vi "Main.vi"(11 "Module Admin":refnum<class "Delacor_lib_QMH_Module Admin.lvclass">) -> ()   [LabVIEW 2026, in "FT-818 CW Key Control.lvlib"]
doc: "This template is based off of the Queued Message Handler design pattern and the Queued Message Handler project template that ships with LabVIEW.\n\nThe main difference is that the queue is private to this module and communication between modules is performed via Broadcast and Request events.\n\nRequest events are wrapped in public API methods and are handled in the Event Handling Loop (EHL) of this VI. Any module can register for Broadcast events sent by this module. The EHL generates messages based on user interface actions.\n\nThe Message Handling Loop (MHL) processes messages generated by the EHL, or by other messages. The messages are string values, so new messages can be added easily to the Message Cases case structure in the MHL. Each message cluster can also provide an optional value for Message Data, which is a variant that can be converted to whatever message-specific data is required.\n_____\nBased on DQMH Dev Tools: Project Template 7.1.2.1547."
uses:
  FT-818 CW Key Control.lvlib
  <vilib>/Delacor/Delacor QMH/Libraries/Message Queue_class/Delacor_lib_QMH_Message Queue.lvclass/Delacor_lib_QMH_Message Queue.ctl
  <vilib>/Delacor/Delacor QMH/Libraries/Module Admin_class/Delacor_lib_QMH_Module Admin.lvclass/Delacor_lib_QMH_Module Admin.ctl
  <vilib>/Delacor/Delacor QMH/Libraries/Message Queue_class/Delacor_lib_QMH_Message Queue.lvclass
  Module Data--cluster.ctl
  <vilib>/Utility/miscctls.llb/LVPointTypeDef.ctl
  <vilib>/Delacor/Delacor QMH/Libraries/Message Queue_class/Delacor_lib_QMH_Enqueue Message (Single).vi
  Stop Argument--cluster.ctl
  <vilib>/Delacor/Delacor QMH/Libraries/Module Admin_class/Delacor_lib_QMH_Module Admin.lvclass
  Connect to radio (Reply Payload)--cluster.ctl
  Connect to radio Argument--cluster.ctl
  <vilib>/Instr/_visa.llb/VISA Configure Serial Port (Instr).vi
  Send CW Tone Argument--cluster.ctl
  Send CW Tone (Reply Payload)--cluster.ctl
  801ab31c-6d94-4327-a799-783b4abf15f8.vi
  0e38ebe7-76c1-4907-b289-0177e71b42e0.vi
panel:
  out "error out":errorcluster
  out "Status":string
  in  "Simulate MHL Error":bool
  in  "Simulate EHL Error":bool
  # "Other processes communicate with this Module via its Public API (wrappers for its Request Events).\n\nThis Module communicates with other processes via its Broadcast Events.\nAny process that wants to receive these messages can register for this module's Broadcast events."
  # "This template is for the DQMH framework. See the block diagram for more information on how to use this template."
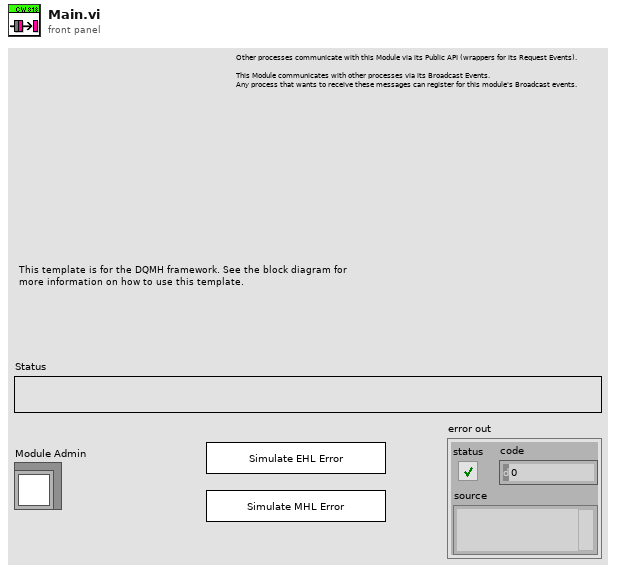
[diagram p1: front panel]
types:
  T1 = typedef "FT-818 CW Key Control.lvlib/Request Events--cluster.ctl" = cluster{"Stop Module":refnum<user-event>, "Show Panel":refnum<user-event>, "Hide Panel":refnum<user-event>, "Get Module Execution Status":refnum<user-event>, "Show Diagram":refnum<user-event>, "Connect to radio":refnum<user-event>, "Send CW Tone":refnum<user-event>}
  T2 = typedef "FT-818 CW Key Control.lvlib/Module Data--cluster.ctl" = cluster{"Status":string, "Radio Comm Port":refnum<visa-resource-name>}
  T3 = enum32{"invalid lock state", "Not Locked", "Locked (No Password)", "Password-protected"}
  T4 = typedef "FT-818 CW Key Control.lvlib/Stop Argument--cluster.ctl" = cluster{"Origin":string, "Exit via Stop Module Req?":bool, "Wait for Module to stop?":bool}
  T5 = typedef "FT-818 CW Key Control.lvlib/Connect to radio Argument--cluster.ctl" = cluster{"Radio Comm Port":refnum<visa-resource-name>, "CAT Rate":u32, "Wait Notifier":refnum<notifier>, "wait for reply":bool}
  T6 = typedef "FT-818 CW Key Control.lvlib/Send CW Tone Argument--cluster.ctl" = cluster{"CW Tone Time (ms)":u32, "Wait Notifier":refnum<notifier>, "wait for reply":bool}
  T7 = typedef "LVPointTypeDef.ctl" = cluster{"Horizontal":i16, "Vertical":i16}
  T8 = enum32{"Invalid", "Standard", "Closed", "Hidden", "Minimized", "Maximized"}
  T9 = typedef "FT-818 CW Key Control.lvlib/Connect to radio (Reply Payload)--cluster.ctl" = cluster{"Connected?":bool, "error":errorcluster}
  T10 = typedef "FT-818 CW Key Control.lvlib/Send CW Tone (Reply Payload)--cluster.ctl" = cluster{"error":errorcluster, "Done?":bool}
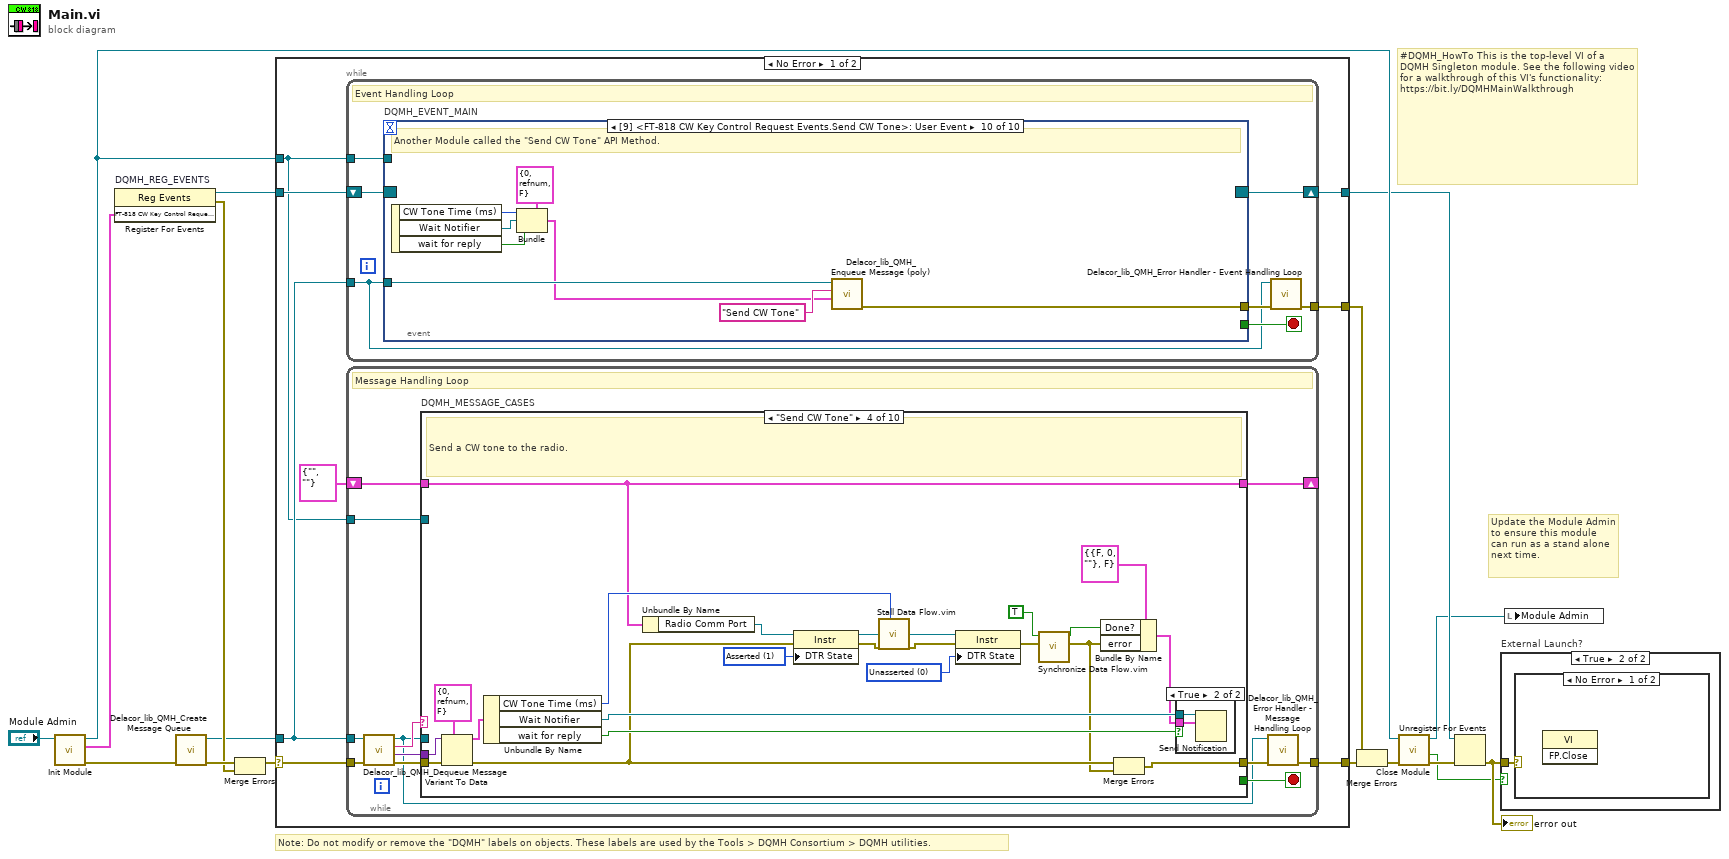
[diagram p0: block diagram]
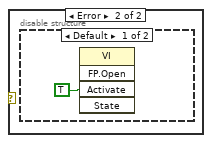
[diagram p3: hidden frame]
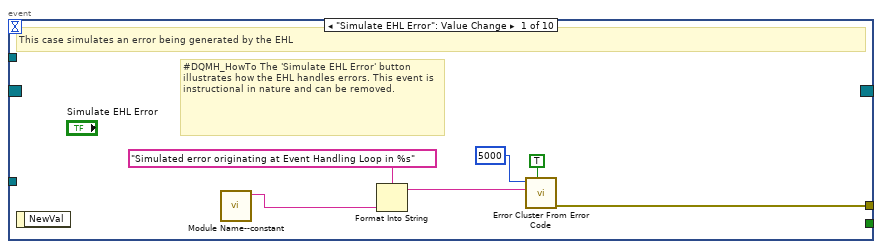
[diagram p5: hidden frame]
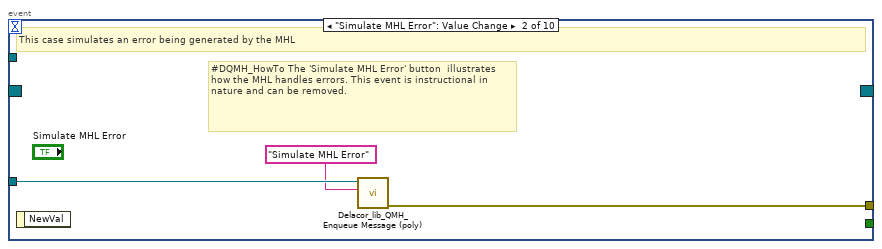
[diagram p6: hidden frame]
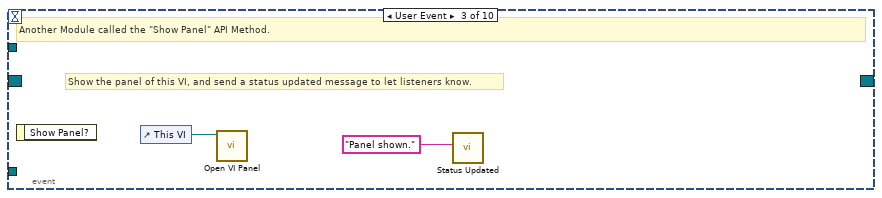
[diagram p7: hidden frame]
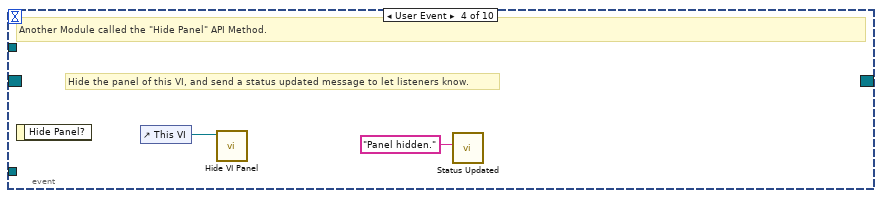
[diagram p8: hidden frame]
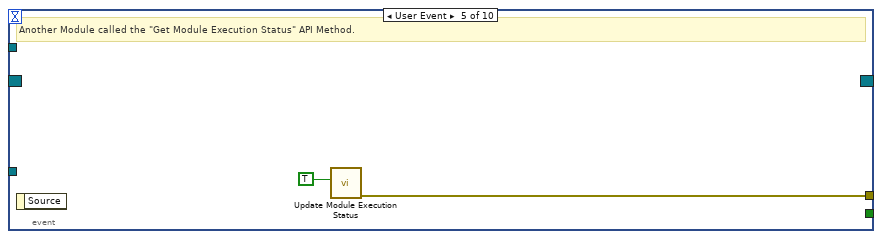
[diagram p9: hidden frame]
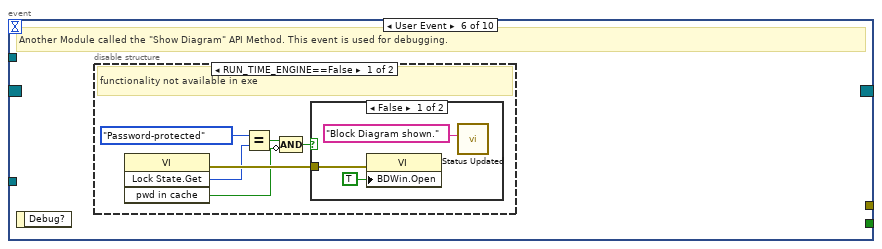
[diagram p10: hidden frame]
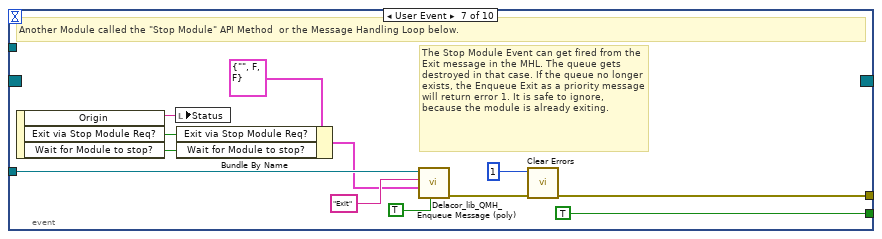
[diagram p13: hidden frame]
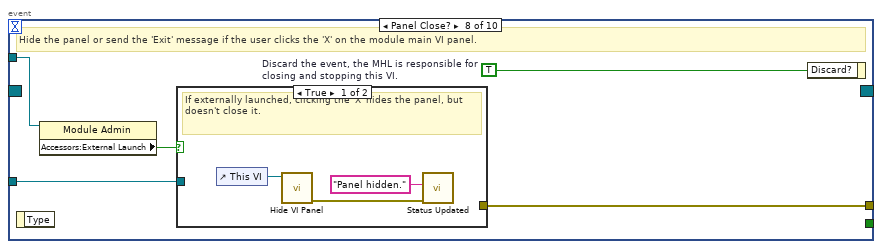
[diagram p14: hidden frame]
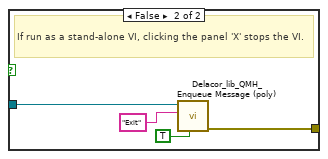
[diagram p15: hidden frame]
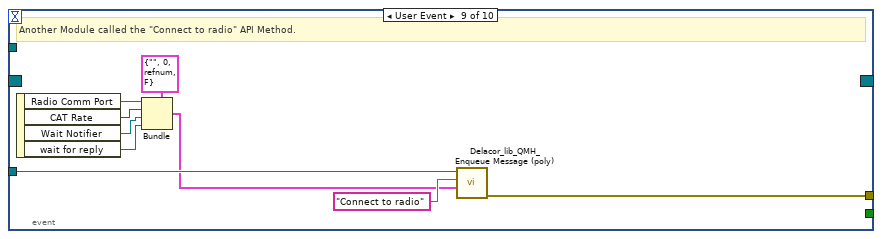
[diagram p16: hidden frame]
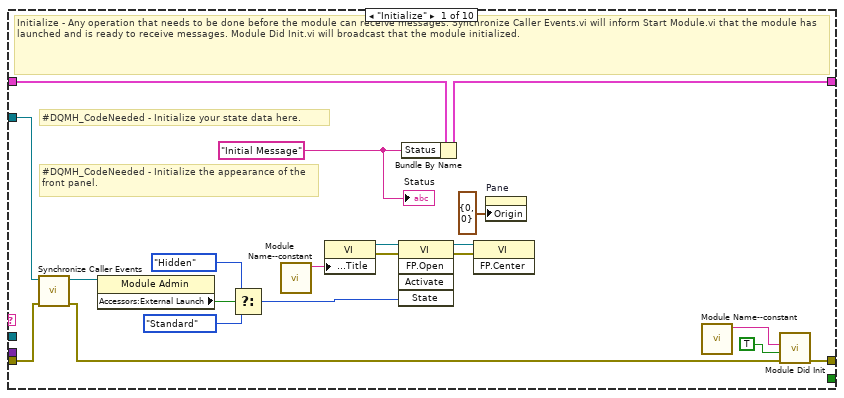
[diagram p17: hidden frame]
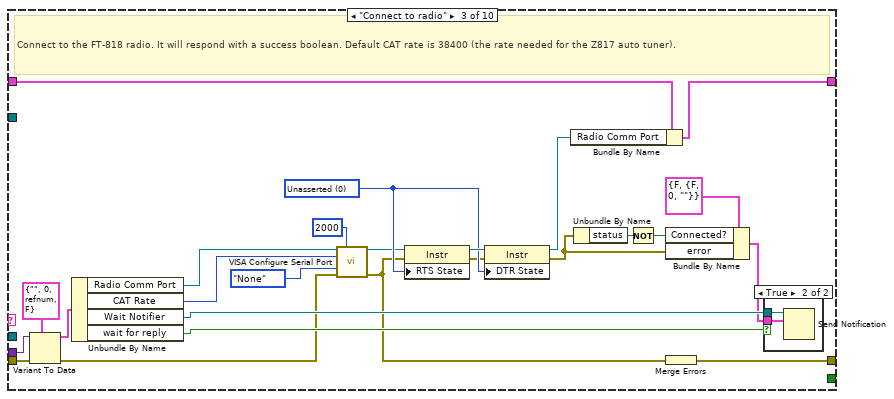
[diagram p19: hidden frame]
diagram:
  # "#DQMH_HowTo This is the top-level VI of a DQMH Singleton module. See the following video for a walkthrough of this VI's functionality: https://bit.ly/DQMHMainWalkthrough"
  # "Note: Do not modify or remove the \"DQMH\" labels on objects. These labels are used by the Tools > DQMH Consortium > DQMH utilities."
  # "Update the Module Admin to ensure this module can run as a stand alone next time."
  n1 = call "Init Module.vi"("Singleton Module Admin in"="Module Admin") -> ("error out"=w16:errorcluster, "FT-818 CW Key Control Request Events"=w5:T1, "Singleton Module Admin out"=w8:refnum<class "Delacor_lib_QMH_Module Admin.lvclass">)  [unwired: 8 in]
  n2 = register-events "DQMH_REG_EVENTS"(w5) -> (reference out=w6:refnum<event-registration>, error out=w9:errorcluster)  [unwired: 2 in]
  n3 = call <vilib>:"Delacor_lib_QMH_Create Message Queue.vi"("error in"=w16) -> ("error out"=w11:errorcluster, "Message Queue"=w4:refnum<class "Delacor_lib_QMH_Message Queue.lvclass">)  [unwired: 9 in]
  n4 = Merge Errors(w11, w9) -> (w10:errorcluster)
  n5 = case shown="No Error" w10 {
    selector: w10 -> [w23 w248]
    tunnel: [w25 w247] -> w17
    tunnel: [w22 w246] -> w7
    tunnel: w6 -> [w20 w246]
    tunnel: w4 -> [w19 w241]
    tunnel: [w24 _] -> w14
    tunnel: w8 -> [w18 w242]
    frame No Error {
      n6 = while {
        tunnel: w19 -> [w26]
        shift-right: [w29] -> w22
        shift-left: w20 -> [w30]
        tunnel: [w31] -> w24
        tunnel: w18 -> [w27]
        stop <- w28 stop-if-true
        # "Event Handling Loop"
        n7 = event "DQMH_EVENT_MAIN" shown="[9] <FT-818 CW Key Control Request Events.Send CW Tone>: User Event" {
          selector: w30 -> [_ _ _ _ _ _ _ _ _ _]
          dyn-events: [_ _ _ _ _ _ _ _ _ _] -> w29
          timeout: _ -> [_ _ _ _ _ _ _ _ _ _]
          tunnel: [_ _ _ _ _ _ TRUE ("Discard?") _ _ _] -> w28
          tunnel: w26 -> [_ w40 _ _ _ _ w64 w71 w89 w97]
          tunnel: [w38 w41 _ _ w47 _ w67 w73 w81 w92] -> w32
          tunnel: w27 -> [_ _ _ _ _ _ _ w70 _ _]
          event "Simulate EHL Error": Value Change {
            # "#DQMH_HowTo The 'Simulate EHL Error' button  illustrates how the EHL handles errors. This event is instructional in nature and can be removed."
            # "This case simulates an error being generated by the EHL"
            n8 = event-data() -> ()  [unwired: 1 in, 1 out]
            n9 = call "Module Name--constant.vi"() -> ("Module Name"=w35:string)  [unwired: 11 in]
            n10 = Format Into String(format string="Simulated error originating at Event Handling Loop in %s", w35) -> (resulting string=w36:string)  [unwired: 2 in, 1 out]
            n11 = call <vilib>:"Error Cluster From Error Code.vi"("show call chain? (False)"=TRUE, "error message (\"\")"=w36, "error code (0)"=5000) -> ("error out"=w38:errorcluster)  [unwired: 6 in]
          }
          event "Simulate MHL Error": Value Change {
            # "#DQMH_HowTo The 'Simulate MHL Error' button  illustrates how the MHL handles errors. This event is instructional in nature and can be removed."
            # "This case simulates an error being generated by the MHL"
            n12 = event-data() -> ()  [unwired: 1 in, 1 out]
            n13 = call-poly <vilib>:"Delacor_lib_QMH_Enqueue Message (poly).vi"("Message"="Simulate MHL Error", "Message Queue in"=w40) -> ("error out"=w41:errorcluster)  [unwired: 8 in, 1 out]
          }
          event User Event {
            # "Show the panel of this VI, and send a status updated message to let listeners know."
            # "Another Module called the \"Show Panel\" API Method."
            n14 = event-data() -> ()  [unwired: 1 in, 1 out]
            n15 = control-ref of="This VI"() -> (w43:refnum<vi>)
            n16 = call "Open VI Panel.vi"("VI"=w43) -> ()  [unwired: 10 in, 1 out]
            n17 = call "Status Updated.vi"("Status"="Panel shown." ("format string")) -> ()  [unwired: 10 in, 1 out]
          }
          event User Event {
            # "Hide the panel of this VI, and send a status updated message to let listeners know."
            # "Another Module called the \"Hide Panel\" API Method."
            n18 = event-data() -> ()  [unwired: 1 in, 1 out]
            n19 = control-ref of="This VI"() -> (w45:refnum<vi>)
            n20 = call "Hide VI Panel.vi"("VI"=w45) -> ()  [unwired: 10 in, 1 out]
            n21 = call "Status Updated.vi"("Status"="Panel hidden." ("format string")) -> ()  [unwired: 10 in, 1 out]
          }
          event User Event {
            # "Another Module called the \"Get Module Execution Status\" API Method."
            n22 = event-data() -> ()  [unwired: 1 in, 1 out]
            n23 = call "Update Module Execution Status.vi"("Running?"=TRUE) -> ("error out"=w47:errorcluster)  [unwired: 10 in]
          }
          event User Event {
            # "Another Module called the \"Show Diagram\" API Method. This event is used for debugging."
            n24 = event-data() -> ()  [unwired: 1 in, 1 out]
            n25 = disable-structure shown="RUN_TIME_ENGINE==False" {
              frame condition #0 (active) {
                # "functionality not available in exe"
                n26 = invoke on="Invoke Node" class="VI" method="Lock State.Get"() -> (error out=w53:errorcluster, "Get Lock State"=w52:T3, "pwd in cache"=w49:bool)  [unwired: 4 in, 1 out]
                n27 = Equal?(x=T3."Password-protected", y=w52) -> (x = y?=w50:bool)
                n28 = Compound Arithmetic op=AND(w50, invert w49) -> (w48:bool)
                n29 = case shown="False" w48 {
                  tunnel: w53 -> [w56 _]
                  frame False {
                    n30 = property on="Property Node" class="VI"(error in=w56, "BDWin.Open"=TRUE ("Block Diagram Window:Open")) -> ()  [unwired: 1 in, 2 out]
                    n31 = call "Status Updated.vi"("Status"="Block Diagram shown." ("format string")) -> ()  [unwired: 10 in, 1 out]
                  }
                  frame True {
                    # "Password-protected VI, and the password is not in the cache. Do not show the diagram."
                  }
                }
              }
              frame condition #1 {
              }
            }
          }
          event User Event {
            # "The Stop Module Event can get fired from the Exit message in the MHL. The queue gets destroyed in that case. If the queue no longer exists, the Enqueue Exit as a priority message will return error 1. It is safe to ignore, because the module is already exiting."
            # "Another Module called the \"Stop Module\" API Method  or the Message Handling Loop below."
            n32 = event-data() -> ("Origin"=w63:string, "Exit via Stop Module Req?"=w59:bool, "Wait for Module to stop?"=w58:bool)  [unwired: 1 in]
            n33 = local write "Status"(w63) -> ()
            n34 = Bundle By Name(cluster=T4 {"Origin"="", "Exit via Stop Module Req?"=FALSE, "Wait for Module to stop?"=FALSE} ("Stop Argument"), "Exit via Stop Module Req?"=w59, "Wait for Module to stop?"=w58) -> (w57:T4)
            n35 = call-poly <vilib>:"Delacor_lib_QMH_Enqueue Message (poly).vi"("Priority Message? (F)"=TRUE, "Message Data"=w57, "Message"="Exit", "Message Queue in"=w64) -> ("error out"=w68:errorcluster)  [unwired: 6 in, 1 out]
            n36 = call <vilib>:"Clear Errors.vi"("error in (no error)"=w68, "specific error code to clear (0: all)"=1) -> ("error out"=w67:errorcluster)  [unwired: 4 in, 1 out]
          }
          event Panel Close? {
            w72 = TRUE  # Discard the event, the MHL is responsible for closing and stopping this VI.
            # "Hide the panel or send the 'Exit' message if the user clicks the 'X' on the module main VI panel."
            n37 = event-data() -> ()  [unwired: 1 in, 1 out]
            n38 = property on="Property Node" class="Module Admin"(reference=w70) -> ("Accessors:External Launch"=w69:bool)  [unwired: 1 in, 2 out]
            n39 = case shown="True" w69 {
              tunnel: w71 -> [_ w79]
              tunnel: [_ w80] -> w73
              frame True {
                # "If externally launched, clicking the 'X' hides the panel, but doesn't close it."
                n40 = control-ref of="This VI"() -> (w76:refnum<vi>)
                n41 = call "Hide VI Panel.vi"("VI"=w76) -> ("error out"=w74:errorcluster)  [unwired: 10 in]
                n42 = call "Status Updated.vi"("error in"=w74, "Status"="Panel hidden." ("format string")) -> ()  [unwired: 9 in, 1 out]
              }
              frame False {
                # "If run as a stand-alone VI, clicking the panel 'X' stops the VI."
                n43 = call-poly <vilib>:"Delacor_lib_QMH_Enqueue Message (poly).vi"("Priority Message? (F)"=TRUE, "Message"="Exit", "Message Queue in"=w79) -> ("error out"=w80:errorcluster)  [unwired: 7 in, 1 out]
              }
            }
            n44 = event-data ("Event Filter Node")("Discard?"=w72) -> ()  [unwired: 1 in, 1 out]
          }
          event User Event {
            # "Another Module called the \"Connect to radio\" API Method."
            n45 = event-data() -> ("Radio Comm Port"=w85:refnum<visa-resource-name>, "CAT Rate"=w84:u32, "Wait Notifier"=w83:refnum<notifier>, "wait for reply"=w82:bool)  [unwired: 1 in]
            n46 = Bundle(cluster=T5 {"Radio Comm Port"="", "CAT Rate"=0, "Wait Notifier"=refnum, "wait for reply"=FALSE} ("Connect to radio Argument"), "Radio Comm Port"=w85, "CAT Rate"=w84, "Wait Notifier"=w83, "wait for reply"=w82) -> (w86:T5)
            n47 = call-poly <vilib>:"Delacor_lib_QMH_Enqueue Message (poly).vi"("Message Data"=w86, "Message"="Connect to radio", "Message Queue in"=w89) -> ("error out"=w81:errorcluster)  [unwired: 7 in, 1 out]
          }
          event User Event {
            # "Another Module called the \"Send CW Tone\" API Method."
            n48 = event-data() -> ("CW Tone Time (ms)"=w93:u32, "Wait Notifier"=w91:refnum<notifier>, "wait for reply"=w90:bool)  [unwired: 1 in]
            n49 = Bundle(cluster=T6 {"CW Tone Time (ms)"=0, "Wait Notifier"=refnum, "wait for reply"=FALSE} ("Send CW Tone Argument"), "CW Tone Time (ms)"=w93, "Wait Notifier"=w91, "wait for reply"=w90) -> (w94:T6)
            n50 = call-poly <vilib>:"Delacor_lib_QMH_Enqueue Message (poly).vi"("Message Data"=w94, "Message"="Send CW Tone", "Message Queue in"=w97) -> ("error out"=w92:errorcluster)  [unwired: 7 in, 1 out]
          }
        }
        n51 = call-dynamic "Delacor_lib_QMH_Error Handler - Event Handling Loop.vi"("error in"=w32, "Message Queue in"=w26) -> ("dup error in"=w31:errorcluster)  [unwired: 8 in, 1 out]
      }
      n52 = while {
        tunnel: w19 -> [w98]
        shift-right: [w106] -> _
        shift-left: T2 {"Status"="", "Radio Comm Port"=""} ("Data Cluster") -> [w107]
        tunnel: w23 -> [w109]
        tunnel: [w101] -> w25
        tunnel: w18 -> [w102]
        stop <- w105 stop-if-true
        # "Message Handling Loop"
        n53 = call-dynamic "Delacor_lib_QMH_Dequeue Message.vi"("error in"=w109, "Message Queue in"=w98) -> ("error out"=w108:errorcluster, "Message Data"=w103:variant, "Message"=w104:string, "Message Queue out"=w99:refnum<class "Delacor_lib_QMH_Message Queue.lvclass">)  [unwired: 6 in]
        n54 = case "DQMH_MESSAGE_CASES" shown="\"Send CW Tone\"" w104 {
          selector: w104 -> [_ _ _ _ _ _ _ _ _ w236]
          tunnel: w99 -> [_ _ _ _ _ _ _ w200 w224 _]
          tunnel: w108 -> [w127 w131 w156 w180 w185 w187 w196 w207 w230 w239]
          tunnel: [w125 w131 w147 w172 w184 w187 w195 w203 w225 w240] -> w100
          tunnel: w107 -> [w116 w130 w155 w164 w183 w186 w193 w202 w216 w237]
          tunnel: [w115 w130 w140 w164 w183 w186 w193 w202 w216 w237] -> w106
          tunnel: [_ _ _ _ _ _ _ _ w223 _] -> w105
          tunnel: w103 -> [_ _ w154 w179 _ _ _ w201 w222 _]
          tunnel: w102 -> [w117 _ _ _ _ _ _ w199 w217 _]
          frame "Initialize" {
            w111 = "Initial Message" ("Initial Message")
            # "#DQMH_CodeNeeded - Initialize the appearance of the front panel."
            # "#DQMH_CodeNeeded - Initialize your state data here."
            # "Initialize - Any operation that needs to be done before the module can receive messages. Synchronize Caller Events.vi will inform Start Module.vi that the module has launched and is ready to receive messages. Module Did Init.vi will broadcast that the module initialized."
            n55 = call "Synchronize Caller Events.vi"("error in"=w127, "Singleton Module Admin in"=w117) -> ("error out"=w126:errorcluster, "Singleton Module Admin out"=w112:refnum<class "Delacor_lib_QMH_Module Admin.lvclass">)  [unwired: 8 in]
            n56 = property on="Property Node" class="Module Admin"(reference=w112) -> ("Accessors:External Launch"=w121:bool)  [unwired: 1 in, 2 out]
            n57 = Select(t=T8."Hidden" ("State"), s=w121, f=T8."Standard" ("State")) -> (s? t:f=w118:T8)
            n58 = call "Module Name--constant.vi"() -> ("Module Name"=w124:string)  [unwired: 11 in]
            n59 = property on="Property Node" class="VI"("Front Panel.Title"=w124) -> (reference out=w123:refnum<vi>, error out=w129:errorcluster)  [unwired: 2 in]
            n60 = invoke on="Invoke Node" class="VI" method="FP.Open"(reference=w123, error in=w129, "State"=w118) -> (reference out=w122:refnum<vi>, error out=w128:errorcluster)  [unwired: 2 in, 3 out]
            n61 = Bundle By Name(cluster=w116, "Status"=w111) -> (w115:T2)
            n62 = invoke on="Invoke Node" class="VI" method="FP.Center"(reference=w122, error in=w128) -> ()  [unwired: 1 in, 3 out]
            n63 = property on="Pane" class="Pane"("Origin"=T7 {"Horizontal"=0, "Vertical"=0}) -> ()  [unwired: 2 in, 2 out]
            n64 = call "Module Name--constant.vi"() -> ("Module Name"=w113:string)  [unwired: 11 in]
            n65 = call "Module Did Init.vi"("error in"=w126, "Initialized?"=TRUE, "Origin"=w113) -> ("error out"=w125:errorcluster)  [unwired: 8 in]
            "Status" <- w111
          }
          frame "---Module Specific---" {
            # "Separator -- The following cases handle messages specific to this Module."
          }
          frame "Connect to radio" {
            w138 = i16 0 items=["Unknown"=-1, "Unasserted"=0, "Asserted"=1] ("Serial Settings:Modem Line Settings:Line RTS State")
            # "Connect to the FT-818 radio. It will respond with a success boolean. Default CAT rate is 38400 (the rate needed for the Z817 auto tuner)."
            n66 = Variant To Data(error in=w156, type=T5 {"Radio Comm Port"="", "CAT Rate"=0, "Wait Notifier"=refnum, "wait for reply"=FALSE} ("Connect to radio Argument"), Variant=w154) -> (data=w152:T5, error out=w144:errorcluster)
            n67 = Unbundle By Name(w152) -> ("Radio Comm Port"=w141:refnum<visa-resource-name>, "CAT Rate"=w146:u32, "Wait Notifier"=w151:refnum<notifier>, "wait for reply"=w150:bool)
            n68 = call-poly "VISA Configure Serial Port"("VISA resource name"=w141, "timeout (10sec)"=u32 2000, "baud rate (9600)"=w146, "parity (0:none)"=enum16{"None", "Odd", "Even", "Mark", "Space"}."None", "error in (no error)"=w144) -> ("VISA resource name out"=w132:refnum<visa-resource-name>, "error out"=w137:errorcluster)  [unwired: 9 in]
            n69 = property class="Instr"(reference=w132, error in=w137, "RTS State"=w138) -> (reference out=w139:refnum<visa-resource-name>, error out=w136:errorcluster)
            n70 = property class="Instr"(reference=w139, error in=w136, "DTR State"=w138) -> (reference out=w134:refnum<visa-resource-name>, error out=w135:errorcluster)
            n71 = Bundle By Name(cluster=w155, "Radio Comm Port"=w134) -> (w140:T2)
            n72 = Unbundle By Name(w135) -> ("status"=w143:bool)
            n73 = Not(x=w143) -> (.not. x?=w142:bool)
            n74 = Bundle By Name(cluster=T9 {"Connected?"=FALSE, "error"={"status"=FALSE, "code"=0, "source"=""}} ("Connect to radio (Reply Payload)"), "Connected?"=w142, "error"=w135) -> (w149:T9)
            n75 = Merge Errors(w137) -> (w147:errorcluster)
            n76 = case "DQMH_FIRE_NOTIFIER" shown="True" w150 {
              tunnel: w151 -> [_ w158]
              tunnel: w149 -> [_ w157]
              frame False {
              }
              frame True {
                n77 = Send Notification(notification=w157, notifier=w158) -> ()  [unwired: 1 in, 2 out]
              }
            }
          }
          frame "Send CW Tone" {
            w168 = i16 0 items=["Unknown"=-1, "Unasserted"=0, "Asserted"=1] ("Serial Settings:Modem Line Settings:Line DTR State")
            w171 = i16 1 items=["Unknown"=-1, "Unasserted"=0, "Asserted"=1] ("Serial Settings:Modem Line Settings:Line DTR State")
            # "Send a CW tone to the radio."
            n78 = Variant To Data(error in=w180, type=T6 {"CW Tone Time (ms)"=0, "Wait Notifier"=refnum, "wait for reply"=FALSE} ("Send CW Tone Argument"), Variant=w179) -> (data=w177:T6, error out=w166:errorcluster)
            n79 = Unbundle By Name(w177) -> ("CW Tone Time (ms)"=w165:u32, "Wait Notifier"=w176:refnum<notifier>, "wait for reply"=w175:bool)
            n80 = Unbundle By Name(w164) -> ("Radio Comm Port"=w163:refnum<visa-resource-name>)
            n81 = property class="Instr"(reference=w163, error in=w166, "DTR State"=w171) -> (reference out=w170:refnum<visa-resource-name>, error out=w167:errorcluster)
            n82 = call "Stall Data Flow.vim"("value in"=w170, "milliseconds to wait"=w165) -> ("value out"=w169:refnum<visa-resource-name>)  [unwired: 1 out]
            n83 = property class="Instr"(reference=w169, error in=w167, "DTR State"=w168) -> (error out=w162:errorcluster)  [unwired: 1 out]
            n84 = call "Synchronize Data Flow.vim"("input 2"=w162, "input 1"=TRUE) -> ("output 2"=w159:errorcluster, "output 1"=w160:bool)  [unwired: 2 in, 2 out]
            n85 = Bundle By Name(cluster=T10 {"error"={"status"=FALSE, "code"=0, "source"=""}, "Done?"=FALSE} ("Send CW Tone (Reply Payload)"), "Done?"=w160, "error"=w159) -> (w174:T10)
            n86 = Merge Errors(w166, w159) -> (w172:errorcluster)
            n87 = case "DQMH_FIRE_NOTIFIER" shown="True" w175 {
              tunnel: w176 -> [_ w182]
              tunnel: w174 -> [_ w181]
              frame False {
              }
              frame True {
                n88 = Send Notification(notification=w181, notifier=w182) -> ()  [unwired: 1 in, 2 out]
              }
            }
          }
          frame "---Copy This Frame---" {
            # "Duplicate this frame when creating new messages.  Change this comment in the duplicated frame to describe this message."
            n89 = Merge Errors(w185) -> (w184:errorcluster)
          }
          frame "---Exit and Error Handling---" {
            # "Separator - The following cases handle errors and exit messages."
          }
          frame "Simulate MHL Error" {
            # "#DQMH_HowTo The 'Simulate MHL Error' button  illustrates how the MHL handles errors. This event is instructional in nature and can be removed."
            # "Simulate an error occurring at the MHL"
            n90 = call "Module Name--constant.vi"() -> ("Module Name"=w189:string)  [unwired: 11 in]
            n91 = Format Into String(format string="Simulated error originating at Message Handling Loop in %s", w189) -> (resulting string=w190:string)  [unwired: 2 in, 1 out]
            n92 = call <vilib>:"Error Cluster From Error Code.vi"("show call chain? (False)"=TRUE, "error message (\"\")"=w190, "error code (0)"=5001) -> ("error out"=w194:errorcluster)  [unwired: 6 in]
            n93 = Merge Errors(w196, w194) -> (w195:errorcluster)
          }
          frame "Error" {
            # "#DQMH_CodeRecommended - If the module is running in standalone mode (External Launch = FALSE), this code will pop up an error dialog and call the 'Exit' message if an error occurs. Add more fine-grained error management here."
            # "Error - Check the error message data and respond accordingly. This message is sent by the \"Error Handler\" VIs at the end of each loop in this application."
            n94 = property on="Property Node" class="Module Admin"(reference=w199) -> ("Accessors:External Launch"=w198:bool)  [unwired: 1 in, 2 out]
            n95 = Variant To Data(error in=w207, type=errorcluster {"status"=FALSE, "code"=0, "source"=""} ("error constant"), Variant=w201) -> (data=w197:errorcluster, error out=w205:errorcluster)
            n96 = local write "error out"(w197) -> ()
            n97 = call "Error Reported.vi"("Error"=w197) -> ()  [unwired: 10 in, 1 out]
            n98 = case shown="False" w198 {
              tunnel: [w212 _] -> w204
              tunnel: w200 -> [w210 _]
              tunnel: w197 -> [w211 _]
              frame False {
                n99 = disable-structure shown="Default" {
                  disable-tunnel: w211 -> [w213 _]
                  frame condition #0 (active) {
                    # "If the module is running standalone, then pop up an error dialog and call the \"Exit\" message."
                    n100 = call <vilib>:"Simple Error Handler.vi"("error in (no error)"=w213) -> ()  [unwired: 4 in, 5 out]
                  }
                  frame condition #1 {
                    # "To prevent the Simple Error Handler VI from being loaded (e.g. when deploying to a Real-Time target), add the Conditional Disable Symbol \"DQMH_Disable_SEH\" to your project and set it to TRUE."
                  }
                }
                n101 = call-poly <vilib>:"Delacor_lib_QMH_Enqueue Message (poly).vi"("Priority Message? (F)"=TRUE, "Message"="Exit", "Message Queue in"=w210) -> ("error out"=w212:errorcluster)  [unwired: 7 in, 1 out]
              }
              frame True {
                # "If the module was launched externally, calling the Error Reported broadcast VI is the only action performed by the \"Error\" message. The module's caller can then process the error appropriately."
              }
            }
            n102 = Merge Errors(w205, w204) -> (w203:errorcluster)
          }
          frame "Exit" {
            w221 = 91  # 91: not all Exit messages will have an argument
            w223 = TRUE  # Stop the VI
            # "Release the message queue reference"
            # "#DQMH_CodeNeeded - Add any required cleanup code here."
            # "Exit - Exit the application."
            n103 = Variant To Data(error in=w230, type=T4 {"Origin"="", "Exit via Stop Module Req?"=FALSE, "Wait for Module to stop?"=FALSE} ("Stop Argument"), Variant=w222) -> (data=w219:T4, error out=w227:errorcluster)
            n104 = call <vilib>:"Clear Errors.vi"("error in (no error)"=w227, "specific error code to clear (0: all)"=w221) -> ("error out"=w229:errorcluster)  [unwired: 4 in, 1 out]
            n105 = control-ref of="This VI"() -> (w218:refnum<vi>)
            n106 = call-dynamic "Delacor_lib_QMH_Release Message Queue.vi"("error in"=w229, "Message Queue"=w224) -> ("error out"=w228:errorcluster)  [unwired: 9 in]
            n107 = call "Handle Exit.vi"("Stop Argument"=w219, "Admin in"=w217, "VI reference"=w218) -> ("error out"=w226:errorcluster)  [unwired: 7 in, 1 out]
            n108 = Unbundle By Name(w216) -> ("Radio Comm Port"=w215:refnum<visa-resource-name>)
            n109 = VISA Close(VISA resource name=w215) -> (error out=w214:errorcluster)  [unwired: 1 in]
            n110 = Merge Errors(w214, w228, w226) -> (w225:errorcluster)
            n111 = call "Error Reported.vi"("Error"=w225) -> ()  [unwired: 10 in, 1 out]
          }
          frame Default {
            # "'Default' case only runs if there is a message that isn't defined in any of the other cases.  Output a programming error."
            n112 = call "Module Name--constant.vi"() -> ("Module Name"=w235:string)  [unwired: 11 in]
            n113 = Format Into String(format string="The invalid message string \"%s\" was received in the Message Handling Loop for module \"%s\".", w236, w235) -> (resulting string=w231:string)  [unwired: 2 in, 1 out]
            n114 = call <vilib>:"Error Cluster From Error Code.vi"("show call chain? (False)"=TRUE, "error message (\"\")"=w231, "error code (0)"=1) -> ("error out"=w238:errorcluster)  [unwired: 6 in]
            n115 = Merge Errors(w239, w238) -> (w240:errorcluster)
          }
        }
        n116 = call-dynamic "Delacor_lib_QMH_Error Handler - Message Handling Loop.vi"("error in"=w100, "Message Queue in"=w99) -> ("dup error in"=w101:errorcluster)  [unwired: 8 in, 1 out]
      }
    }
    frame Error {
      # "Synchronize Caller Events.vi will inform Start Module.vi that the module has launched and will let the code calling Start Module.vi register for broadcasts and would permit the caller receive the broadcast that an error occurred at launch time."
      n117 = call-dynamic "Delacor_lib_QMH_Release Message Queue.vi"("error in"=w248, "Message Queue"=w241) -> ("error out"=w247:errorcluster)  [unwired: 9 in]
      n118 = call "Synchronize Caller Events.vi"("Singleton Module Admin in"=w242) -> ("error out"=w249:errorcluster)  [unwired: 9 in, 1 out]
      n119 = call "Module Name--constant.vi"() -> ("Module Name"=w245:string)  [unwired: 11 in]
      n120 = Format Into String(format string="An error occurred during initialization. %s is no longer running.", w245) -> (resulting string=w243:string)  [unwired: 2 in, 1 out]
      n121 = Merge Errors(w247, w249) -> (w250:errorcluster)
      n122 = call "Error Reported.vi"("Additional Information"=w243, "Error"=w250) -> ()  [unwired: 9 in, 1 out]
    }
  }
  n123 = Merge Errors(w14, w17) -> (w13:errorcluster)
  n124 = call "Close Module.vi"("error in"=w13, "Module Admin in"=w8) -> ("error out"=w15:errorcluster, "External Launch"=w1:bool, "Module Admin out"=w2:refnum<class "Delacor_lib_QMH_Module Admin.lvclass">)  [unwired: 7 in]
  n125 = Unregister For Events(event registration refnum=w7, error in=w15) -> (error out=w12:errorcluster)
  "error out" <- w12
  n126 = case "External Launch?" shown="True" w1 {
    tunnel: w12 -> [_ w251]
    frame False {
    }
    frame True {
      n127 = case shown="No Error" w251 {
        frame No Error {
          n128 = invoke on="Invoke Node" class="VI" method="FP.Close"() -> ()  [unwired: 3 in, 3 out]
        }
        frame Error {
          n129 = disable-structure shown="Default" {
            frame condition #0 (active) {
              n130 = invoke class="VI" method="FP.Open"("Activate"=TRUE ("Activate?")) -> ()  [unwired: 4 in, 5 out]
            }
            frame condition #1 {
              # "Don't show panel on error if running inside a built EXE."
            }
          }
        }
      }
    }
  }
  n131 = local write "Module Admin"(w2) -> ()
